vi "Display Elapse Time.vi"(10 "Reset?":bool caption="Reset", 11 "Game Board in":refnum<class "Game Board.lvclass">) -> (2 "Time has Elapsed?":bool caption="Time has Elapsed")   [LabVIEW 2024, in "Game Board.lvclass"]
doc: "MIT Licence\nCopyright (c) 2024 David Grollier"
uses:
  Game Board.lvclass
  Game Board.lvclass/Game Board.ctl
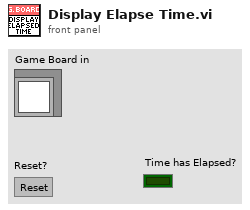
[diagram p1: front panel]
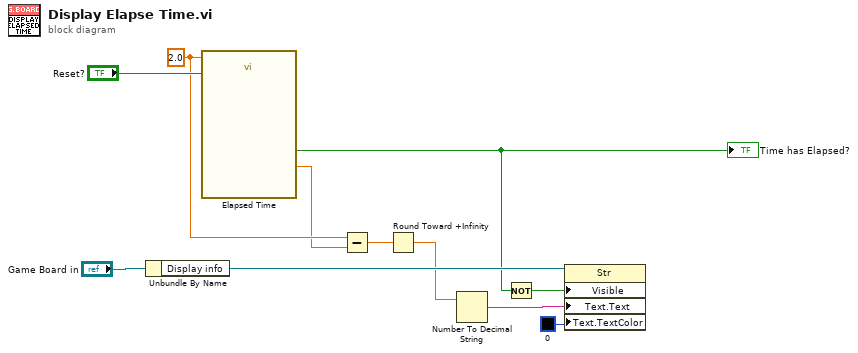
[diagram p0: block diagram]
diagram:
  w7 = 2.0 ("Time Target (s)")
  n1 = Unbundle By Name("Game Board in") -> ("Display info"=w9:refnum<vi>)
  n2 = call "Elapsed Time"("Time Target (s)"=w7, "Reset"="Reset?") -> ("Elapsed Time (s)"=w6:dbl, "Time has Elapsed"=w8:bool)  [unwired: 10 in, 6 out]
  "Time has Elapsed?" <- w8
  n3 = Subtract(x=w7, y=w6) -> (x-y=w5:dbl)
  n4 = Round Toward +Infinity(x=w5) -> (ceil(x): smallest int >= x=w4:dbl)
  n5 = Number To Decimal String(number=w4) -> (decimal integer string=w1:string)  [unwired: 1 in]
  n6 = Not(x=w8) -> (.not. x?=w2:bool)
  n7 = property class="Str"(reference=w9, "Visible"=w2, "Text.Text"=w1, "Text.TextColor"=u32 0 ("Text.Text Colors:Text Color")) -> ()  [unwired: 1 in, 2 out]
